vi "Memory.Array.Numeric.Read power of 2.vi"(8 "error in (no error)":errorcluster, 11 "Numeric Array in":refnum<class "Memory.Array.Numeric.lvclass">) -> (0 "error out":errorcluster, 2 "power of 2":i16, 3 "Numeric Array out":refnum<class "Memory.Array.Numeric.lvclass">)   [LabVIEW 2016, in "LabVIEW Memory Manager.lvlib" / "Memory.Array.Numeric.lvclass"]
uses:
  Memory.Array.Numeric.lvclass
  Memory.Array.Numeric.lvclass/Memory.Array.Numeric.ctl
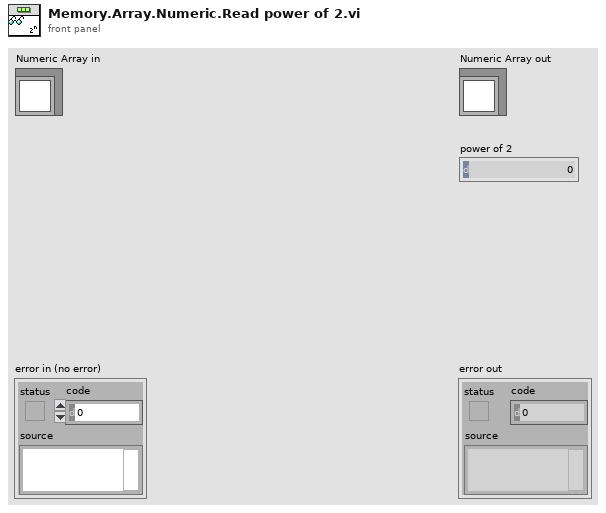
[diagram p1: front panel]
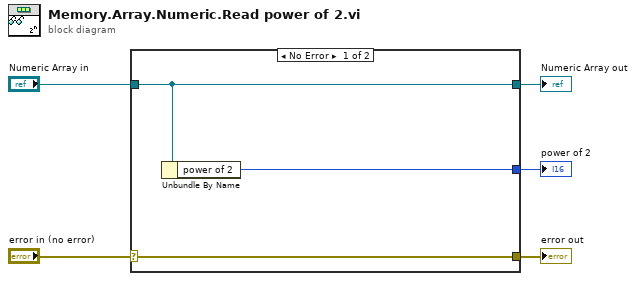
[diagram p0: block diagram]
diagram:
  n1 = case shown="No Error" "error in (no error)" {
    selector: "error in (no error)" -> [w8 w9]
    tunnel: [w8 w9] -> w4
    tunnel: [w7 w10] -> w2
    tunnel: "Numeric Array in" -> [w7 w10]
    tunnel: [w6 _] -> w1
    frame No Error {
      n2 = Unbundle By Name(w7) -> ("power of 2"=w6:i16)
    }
    frame Error {
    }
  }
  "error out" <- w4
  "Numeric Array out" <- w2
  "power of 2" <- w1
